vi "CLD 15 FGV for Text String Parsing Solution.vi"(8 "Fehler (Eingang)":T2, 11 "Modus":T3) -> (0 "Fehler (Ausgang)":T2)   [LabVIEW 2009]
doc: "CLD 15 - In dieser Zusatzaufgabe wird eine FGV auf Grundlage der CLD-Lösung 15 erstellt. Mit diesem VI werden die Datei ausgelesen. Die Daten der Datei werden mit Hilfe von zwei Sub-VIs für die weitere Verwendung analysiert und anschließend formatiert."
uses:
  CLD 15 CSV file data structure.ctl
  <vilib>/Utility/file.llb/Write To Spreadsheet File (string).vi
  <vilib>/Utility/file.llb/Read From Spreadsheet File (string).vi
  CLD 15 CSV file enum.ctl
panel:
  out "Formatierte Daten (Ausgang)":T1[](array[typedef])
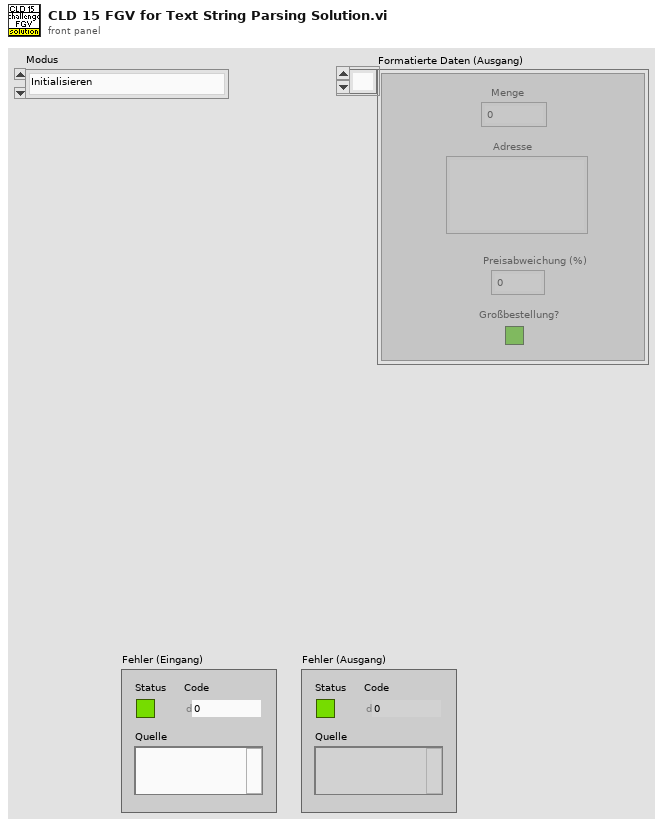
[diagram p1: front panel]
types:
  T1 = typedef "CLD 15 CSV file data structure.ctl" = cluster{"Menge":i32, "Adresse":string, "Preisabweichung (%)":dbl, "Großbestellung?":bool}
  T2 = cluster{"Status":bool, "Code":i32, "Quelle":string}
  T3 = typedef "CLD 15 CSV file enum.ctl" = enum16{"Initialisieren", "CSV lesen", "Daten verarbeiten", "CSV schreiben"}
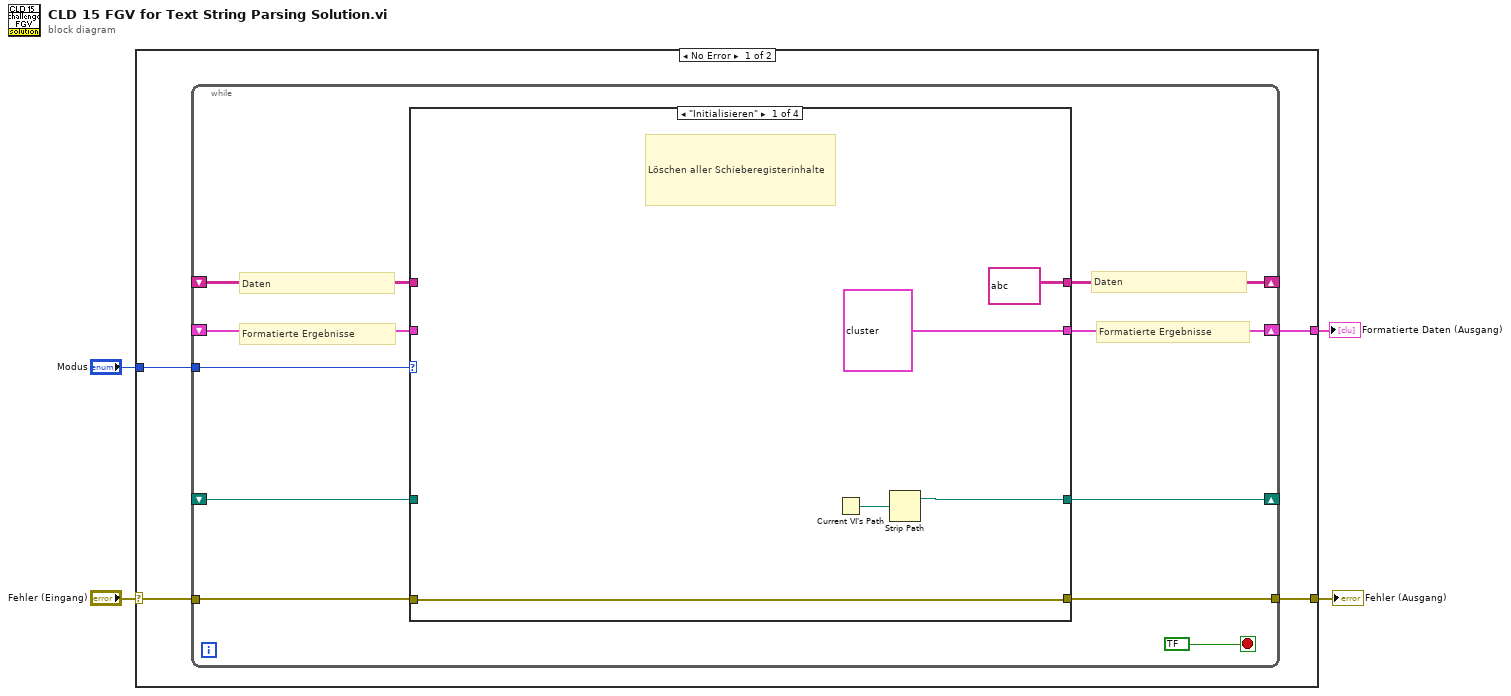
[diagram p0: block diagram]
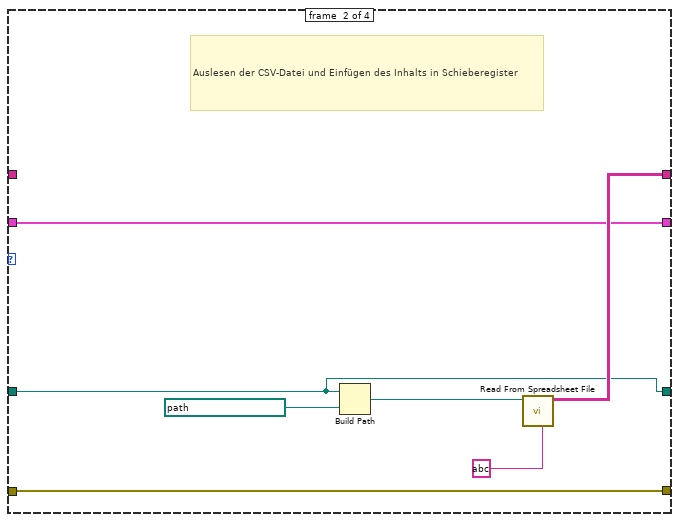
[diagram p2: hidden frame]
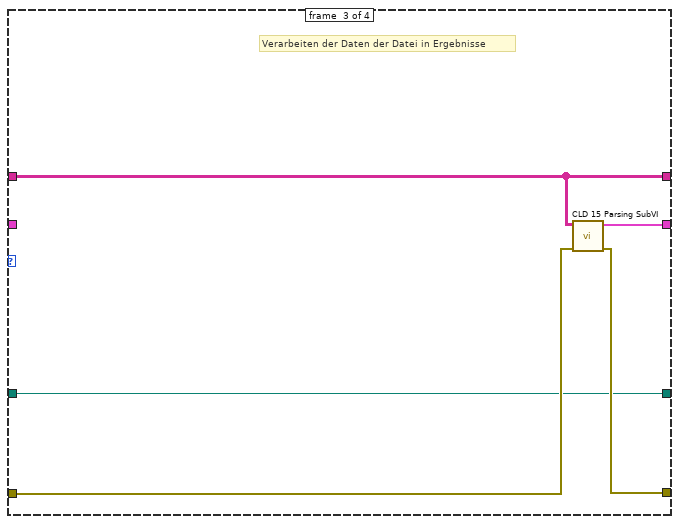
[diagram p3: hidden frame]
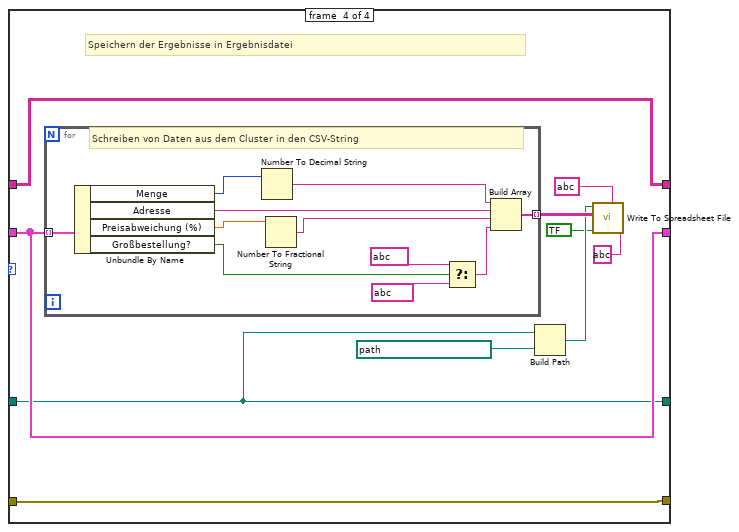
[diagram p4: hidden frame]
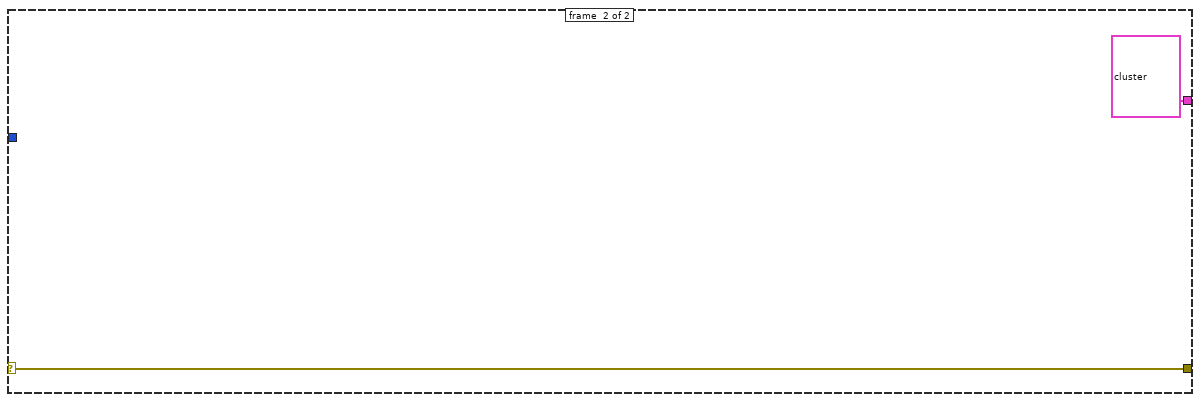
[diagram p5: hidden frame]
diagram:
  n1 = case shown="No Error" "Fehler (Eingang)" {
    selector: "Fehler (Eingang)" -> [w6 w58]
    tunnel: [w8 T1[] ? ("[Daten, Eingang]")] -> w1
    tunnel: "Modus" -> [w7 _]
    tunnel: [w5 w58] -> w2
    frame #0 {
      n2 = while {
        tunnel: w7 -> [w17]
        tunnel: w6 -> [w16]
        tunnel: [w15] -> w5
        shift-right: [w18] -> w8
        shift-left: _ -> [w13]
        shift-right: [w12] -> _
        shift-left: _ -> [w11]
        shift-right: [w10] -> _
        shift-left: _ -> [w9]
        stop <- bool ? stop-if-true
        # "Formatierte Ergebnisse"
        # "Daten"
        # "Formatierte Ergebnisse"
        # "Daten"
        n3 = case shown="\"Initialisieren\"" w17 {
          tunnel: w9 -> [_ w24 w31 w36]
          tunnel: [T1[] ? ("Daten (Eingang)") w27 w34 w38] -> w18
          tunnel: w16 -> [w21 w28 w33 w39]
          tunnel: [w21 w28 w32 w39] -> w15
          tunnel: w13 -> [_ w27 _ w38]
          tunnel: [string[][] ? ("Alle Zeilen") w29 w35 w37] -> w12
          tunnel: w11 -> [_ _ w35 w37]
          tunnel: [w19 w24 w31 w36] -> w10
          frame #0 {
            # "Löschen aller Schieberegisterinhalte"
            n4 = Current VI's Path() -> (path=w20:path)
            n5 = Strip Path(path=w20) -> (stripped path=w19:path)  [unwired: 1 out]
          }
          frame #1 {
            # "Auslesen der CSV-Datei und Einfügen des Inhalts in Schieberegister"
            n6 = Build Path(base path=w24, name or relative path=path ?) -> (appended path=w25:path)
            n7 = call-poly <vilib>:"Read From Spreadsheet File.vi"("delimiter (\\t)"=string ? ("Trennzeichen (\\t)"), "file path (dialog if empty)"=w25) -> ("all rows"=w29:string[][])  [unwired: 5 in, 4 out]
          }
          frame #2 {
            # "Verarbeiten der Daten der Datei in Ergebnisse"
            n8 = call "CLD 15 Parsing SubVI.vi"("Fehler (Eingang)"=w33, "Alle Zeilen (Eingang)"=w35) -> ("Fehler (Ausgang)"=w32:T2, "Daten (Ausgang)"=w34:T1[])  [unwired: 8 in]
          }
          frame #3 {
            # "Speichern der Ergebnisse in Ergebnisdatei"
            n9 = for {
              tunnel: [w47] -> w45 mode=indexing
              tunnel: w38 -> [w46] mode=indexing
              # "Schreiben von Daten aus dem Cluster in den CSV-String"
              n10 = Unbundle By Name(w46) -> ("Menge"=w56:i32, "Adresse"=w50:string, "Preisabweichung (%)"=w55:dbl, "Großbestellung?"=w54:bool)
              n11 = Number To Decimal String(number=w56) -> (decimal integer string=w51:string)  [unwired: 1 in]
              n12 = Number To Fractional String(number=w55) -> (F-format string=w49:string)  [unwired: 3 in]
              n13 = Select(t=string ?, s=w54, f=string ?) -> (s? t:f=w48:string)
              n14 = Build Array(w51, w50, w49, w48) -> (w47:string[])
            }
            n15 = Build Path(base path=w36, name or relative path=path ?) -> (appended path=w41:path)
            n16 = call-poly <vilib>:"Write To Spreadsheet File.vi"("delimiter (\\t)"=string ? ("Trennzeichen (\\t)"), "format (%s)"=string ? ("Format (%s)"), "append to file? (new file:F)"=bool ? ("An Datei anhängen? (Neue Datei:F)"), "2D data"=w45, "file path (dialog if empty)"=w41) -> ()  [unwired: 3 in, 1 out]
          }
        }
      }
    }
    frame #1 {
    }
  }
  "Fehler (Ausgang)" <- w2
  "Formatierte Daten (Ausgang)" <- w1
